vi "IS Open Connection.vi"(8 "error in (no error)":errorcluster, 11 "Access Key":string) -> (0 "error out":errorcluster, 3 "IS Session":T1)   [LabVIEW 2018]
doc: "This VI opens a new HTTP Request with the Initial State API. You provide your Initial State Access Key and receive an active Initial State session with proper headers already set."
uses:
  Controls/IS Session.ctl
  <vilib>/httpClient/ClientHandle.ctl
  <vilib>/httpClient/LabVIEWHTTPClient.lvlib
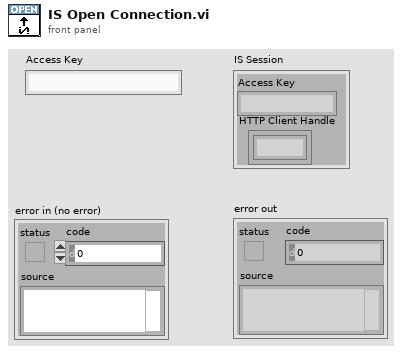
[diagram p1: front panel]
types:
  T1 = typedef "IS Session.ctl" = cluster{"Access Key":string, "HTTP Client Handle":T2}
  T2 = typedef "LabVIEWHTTPClient.lvlib/ClientHandle.ctl" = refnum<k1>
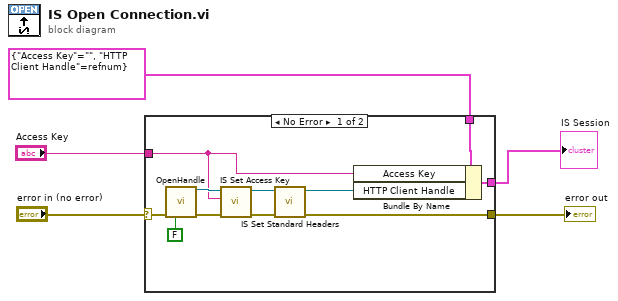
[diagram p0: block diagram]
diagram:
  n1 = case shown="No Error" "error in (no error)" {
    selector: "error in (no error)" -> [w16 w18]
    tunnel: [w7 w18] -> w5
    tunnel: "Access Key" -> [w11 _]
    tunnel: [w15 w17] -> w2
    tunnel: T1 {"Access Key"="", "HTTP Client Handle"=refnum} ("IS Session") -> [w14 w17]
    frame No Error {
      n2 = call <vilib>:"OpenHandle.vi"("error in (no error)"=w16, "verify server(true)"=FALSE) -> ("client handle out"=w13:T2, "error out"=w12:errorcluster)  [unwired: 12 in]
      n3 = call "IS Set Access Key.vi"("HTTP Client Handle in"=w13, "Access Key"=w11, "error in (no error)"=w12) -> ("HTTP Client Handle out"=w10:T2, "error out"=w9:errorcluster)  [unwired: 6 in]
      n4 = call "IS Set Standard Headers.vi"("error in (no error)"=w9, "client handle"=w10) -> ("error out"=w7:errorcluster, "client handle out"=w8:T2)  [unwired: 8 in]
      n5 = Bundle By Name(cluster=w14, "Access Key"=w11, "HTTP Client Handle"=w8) -> (w15:T1)
    }
    frame Error {
    }
  }
  "error out" <- w5
  "IS Session" <- w2
